vi "Y Stage Module.vi"(7 "Set/Get":T2=enum."Get", 8 "Error In":errorcluster, 10 "Action":T3=enum."Stop", 11 "Cluster In":T1={"Device SN"="45876539", "Is.Connected?"=FALSE, "Is.Enabled?"=FALSE, "Position"=0.0, "AccelerationMaximum"=0.0, "VelocityMaximum"=0.0, "Acceleration"=0.0, "Velocity"=0.0, "waitTimeout (ms)"=0}) -> (0 "Error Out":errorcluster, 3 "Cluster Out":T1={"Device SN"="45876539", "Is.Connected?"=FALSE, "Is.Enabled?"=FALSE, "Position"=0.0, "AccelerationMaximum"=0.0, "VelocityMaximum"=0.0, "Acceleration"=0.0, "Velocity"=0.0, "waitTimeout (ms)"=0})   [LabVIEW 2014]
uses:
  Test Code/Hardware/Translation Stage/Ctrls/Motion Translation Module Control.ctl
  Test Code/Hardware/Translation Stage/Ctrls/Translation Stage Cluster.ctl
  Test Code/General/Controls/Set Get Controls.ctl
  C:/Projects/Serial Sectioning OCT - TortoiseGIT/SerialSectOCT/Software/Test Code/Thorlabs.MotionControl.Controls.dll
  Test Code/Thorlabs.MotionControl.Controls.dll
panel:
  in  "LTS Reference":refnum<k24>(container)
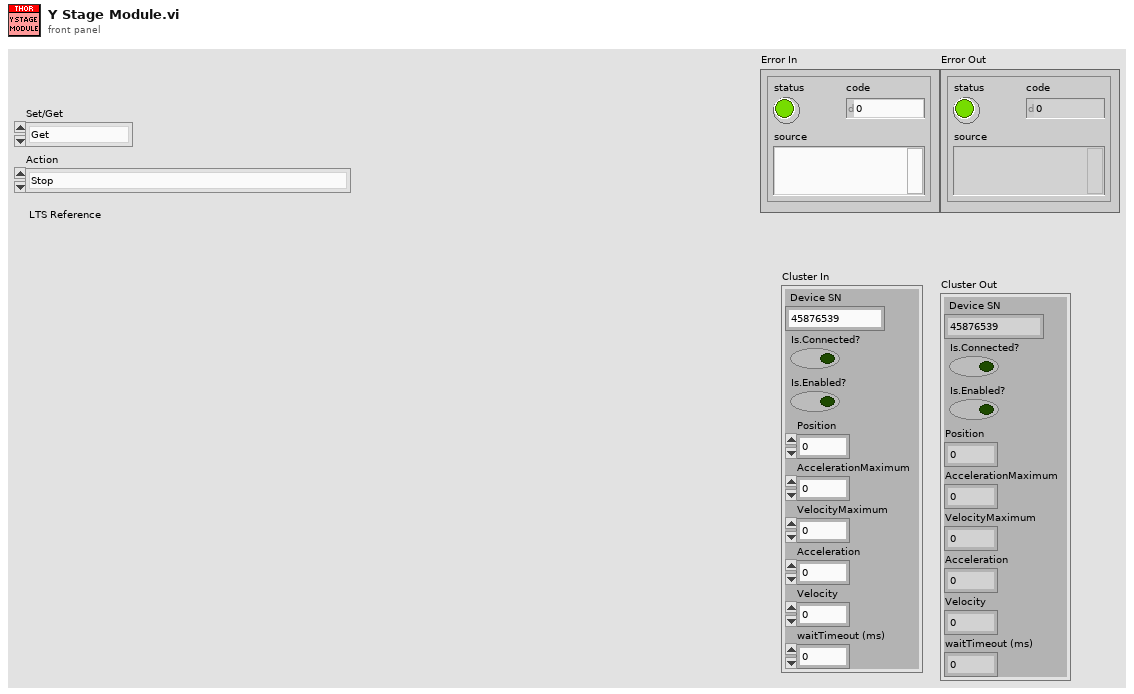
[diagram p1: front panel]
types:
  T1 = typedef "Translation Stage Cluster.ctl" = cluster{"Device SN":string, "Is.Connected?":bool, "Is.Enabled?":bool, "Position":dbl, "AccelerationMaximum":dbl, "VelocityMaximum":dbl, "Acceleration":dbl, "Velocity":dbl, "waitTimeout (ms)":i32}
  T2 = typedef "Set Get Controls.ctl" = enum16{"Set", "Get"}
  T3 = typedef "Motion Translation Module Control.ctl" = enum16{"Init", "Home", "Configure", "Velocity/Accel", "Position", "Jog", "Stop", "Uninit"}
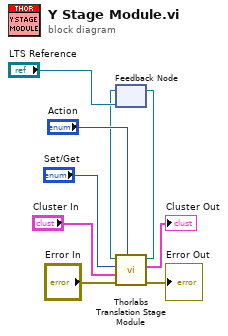
[diagram p0: block diagram]
diagram:
  n1 = feedback #1("LTS Reference") -> (w1:refnum<k24>)
  n2 = call "Thorlabs Translation Stage Module.vi"("Action"="Action", "error in (no error)"="Error In", "Cluster In"="Cluster In", "Set/Get"="Set/Get", ".NET Refnum in"=w1) -> ("error out"=→"Error Out":errorcluster, "Cluster out"=→"Cluster Out":T1, ".NET Refnum out"=w3:refnum<k24>)  [unwired: 4 in]
  n3 = feedback-in #1(w3) -> ()
